vi "RemoteControl_Create.vi"(8 "error in (no error)":errorcluster, 11 "reference in":refnum<class "RemoteControl.lvclass">) -> (0 "error out":errorcluster, 3 "reference out":refnum<class "RemoteControl.lvclass">)   [LabVIEW 2012, in "RemoteControl.lvclass"]
uses:
  RemoteControl.lvclass
  Command_class/Command.lvclass
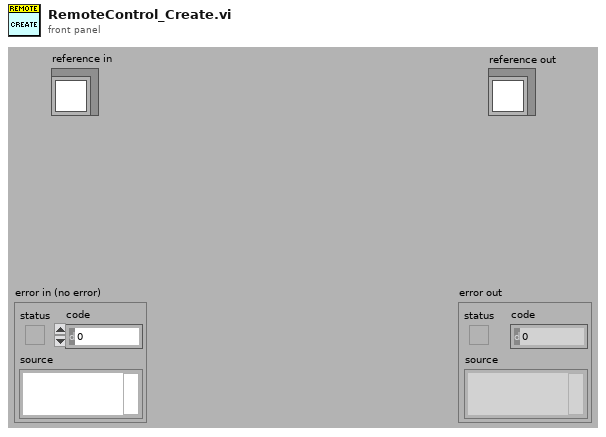
[diagram p1: front panel]
types:
  T1 = typedef "RemoteControl.lvclass/ObjectAttributes.ctl" = cluster{"OnCommands":refnum<class "Command.lvclass">[], "OffCommands":refnum<class "Command.lvclass">[], "UndoCommand":refnum<class "Command.lvclass">}
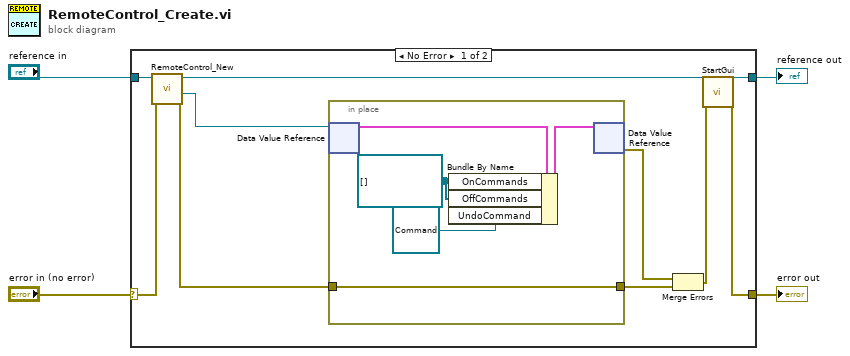
[diagram p0: block diagram]
diagram:
  n1 = case shown="No Error" "error in (no error)" {
    selector: "error in (no error)" -> [w13 w21]
    tunnel: [w5 w21] -> w3
    tunnel: "reference in" -> [w14 w20]
    tunnel: [w7 w20] -> w1
    frame No Error {
      n2 = call "RemoteControl_New.vi"("error in (no error)"=w13, "reference in"=w14) -> ("error out"=w10:errorcluster, "DVRRefOut"=w11:refnum<data-value>, "reference out"=w8:refnum<class "RemoteControl.lvclass">)  [unwired: 6 in, 1 out]
      n3 = in-place {
        in-place-border: w10 -> [w17]
        in-place-border: [w17] -> w9
        w16 = refnum<class "Command.lvclass">[] [] ("OnCommands")
        n4 = in-place-dvr #1(w11) -> (w18:T1)  [unwired: 1 out]
        n5 = Bundle By Name(cluster=w18, "OnCommands"=w16, "OffCommands"=w16, "UndoCommand"=refnum<class "Command.lvclass"> refnum) -> (w19:T1)
        n6 = in-place-dvr #1(w19) -> (w12:errorcluster)  [unwired: 1 out]
      }
      n7 = Merge Errors(w12, w9) -> (w6:errorcluster)
      n8 = call "StartGui.vi"("reference in"=w8, "error in (no error)"=w6) -> ("reference out"=w7:refnum<class "RemoteControl.lvclass">, "error out"=w5:errorcluster)  [unwired: 14 in, 2 out]
    }
    frame Error {
    }
  }
  "error out" <- w3
  "reference out" <- w1
